vi "analyze magnet.vi"(0 "display queues":T3, 1 "disk queues":T3, 3 "trigger":bool, 4 "graph type":enum16{"absolute", "relative"}(ring), 5 "error in (no error)":errorcluster, 11 "toffset":dbl, 12 "crossing stats":T2) -> (10 "mag pos axes limits":cluster{"mag pos max":dbl, "mag pos min":dbl}, 14 "x-y magnet graph":cluster{sgl[], sgl[]}[](array[cluster]), 15 "magnet time graphs":cluster{dbl[], sgl[]}[](array[cluster]), 16 "fit parameters":T1, 19 "error out":errorcluster)   [LabVIEW 2017]
uses:
  typedefs/queue cluster.ctl
  typedefs/reading queue.ctl
  typedefs/reading.ctl
  typedefs/readingType.ctl
  typedefs/reading 1 queue.ctl
  typedefs/reading1.ctl
  typedefs/magnetic field fit.ctl
panel:
  in  "time range (s)":dbl=2.2 format="%#_13g"
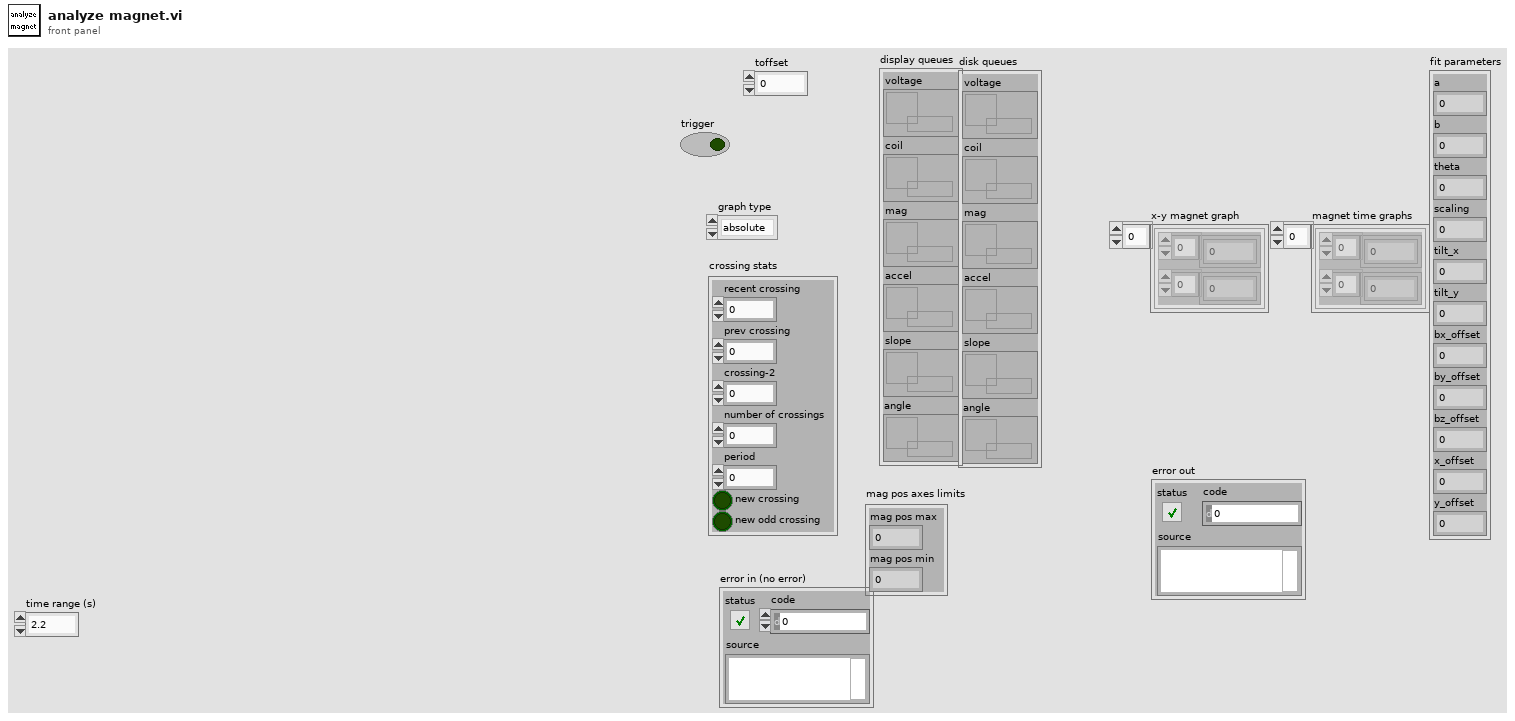
[diagram p1: front panel]
types:
  T1 = typedef "magnetic field fit.ctl" = cluster{"a":dbl, "b":dbl, "theta":dbl, "scaling":dbl, "tilt_x":dbl, "tilt_y":dbl, "bx_offset":dbl, "by_offset":dbl, "bz_offset":dbl, "x_offset":dbl, "y_offset":dbl}
  T2 = cluster{"recent crossing":dbl, "prev crossing":dbl, "crossing-2":dbl, "number of crossings":i32, "period":dbl, "new crossing":bool, "new odd crossing":bool}
  T3 = typedef "queue cluster.ctl" = cluster{"voltage":T4, "coil":T4, "mag":T4, "accel":T4, "slope":T5, "angle":T4}
  T4 = typedef "reading queue.ctl" = refnum<queue>
  T5 = typedef "reading 1 queue.ctl" = refnum<queue>
  T6 = typedef "reading.ctl" = cluster{"reading type":T7, "time":fxp<+,48,48>, "x":sgl, "y":sgl, "z":sgl, "XSUM":u8}
  T7 = typedef "readingType.ctl" = enum8{"SYNC", "DETVAL", "COILI", "MAGVEC", "ACCVEC"}
  T8 = cluster{"tx":cluster{dbl[], sgl[]}, "ty":cluster{dbl[], sgl[]}, "tz":cluster{dbl[], sgl[]}, "xy":cluster{sgl[], sgl[]}}
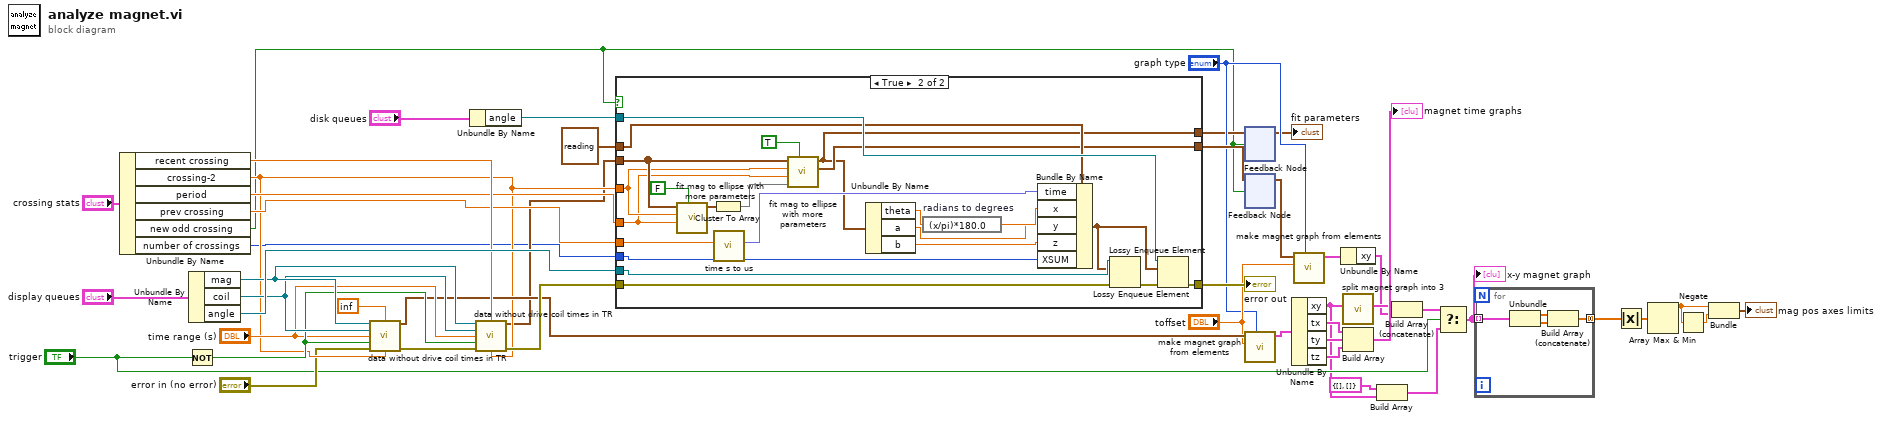
[diagram p0: block diagram]
diagram:
  n1 = Unbundle By Name("crossing stats") -> ("recent crossing"=w41:dbl, "crossing-2"=w31:dbl, "period"=w32:dbl, "prev crossing"=w33:dbl, "new odd crossing"=w16:bool, "number of crossings"=w3:i32)
  n2 = Not(x="trigger") -> (.not. x?=w38:bool)
  n3 = Unbundle By Name("display queues") -> ("mag"=w40:T4, "coil"=w39:T4, "angle"=w46:T4)
  n4 = call "data without drive coil times in TR.vi"("data"=w40, "t1"=inf, "coil"=w39, "recent interval"="time range (s)", "most recent?"=w38, "error in (no error)"="error in (no error)", "t0"=w31) -> ("data_no_coil"=w35:T6[], "error out"=w18:errorcluster)  [unwired: 6 in, 1 out]
  n5 = Unbundle By Name("disk queues") -> ("angle"=w42:T4)
  n6 = call "data without drive coil times in TR.vi"("data"=w40, "t1"=w41, "coil"=w39, "recent interval"="time range (s)", "most recent?"=w38, "error in (no error)"=w18, "t0"=w31) -> ("data_no_coil"=w30:T6[], "error out"=w44:errorcluster)  [unwired: 6 in, 1 out]
  n7 = case shown="True" w16 {
    tunnel: w46 -> [_ w72]
    tunnel: [w49 w69] -> w45
    tunnel: w44 -> [w49 w71]
    tunnel: w42 -> [_ w68]
    tunnel: T6 {"reading type"=enum."SYNC", "time"=0.0, "x"=0.0, "y"=0.0, "z"=0.0, "XSUM"=0} ("angle and time") -> [_ w67]
    tunnel: w33 -> [_ w64]
    tunnel: w32 -> [_ w53]
    tunnel: w31 -> [_ w54]
    tunnel: w30 -> [_ w55]
    tunnel: [_ w57] -> w29
    tunnel: [_ w56] -> w17
    tunnel: w3 -> [_ w62]
    frame False {
    }
    frame True {
      n8 = call "fit mag to ellipse with more parameters.vi"("advanced fit"=FALSE, "T"=w53, "t0"=w54, "mag no drive"=w55) -> ("fit parameters"=w52:T1)  [unwired: 5 in, 2 out]
      n9 = Cluster To Array(cluster=w52) -> (array=w51:dbl[])
      n10 = call "time s to us.vi"("time (s)"=w64) -> ("time (us)"=w63:fxp<+,48,48>)  [unwired: 10 in]
      n11 = call "fit mag to ellipse with more parameters.vi"("advanced fit"=TRUE, "starting parameters"=w51, "T"=w53, "t0"=w54, "mag no drive"=w55) -> ("fit magnetic field"=w57:T6[], "fit parameters"=w56:T1)  [unwired: 4 in, 1 out]
      n12 = Unbundle By Name(w56) -> ("theta"=w65:dbl, "a"=w60:dbl, "b"=w59:dbl)
      n13 = expression code="(x/pi)*180.0" "radians to degrees"(w65) -> (w61:dbl)
      n14 = Bundle By Name(cluster=w67, "time"=w63, "x"=w61, "y"=w60, "z"=w59, "XSUM"=w62) -> (w66:T6)
      n15 = Lossy Enqueue Element(queue=w72, element=w66, error in (no error)=w71) -> (error out=w70:errorcluster)  [unwired: 3 out]
      n16 = Lossy Enqueue Element(queue=w68, element=w66, error in (no error)=w70) -> (error out=w69:errorcluster)  [unwired: 3 out]
    }
  }
  "error out" <- w45
  n17 = feedback #1() -> (→"fit parameters":T1)  [unwired: 1 in]
  n18 = feedback-in #1(w17, w16) -> ()
  n19 = feedback-in #2(w29, w16) -> ()
  n20 = feedback #2() -> (w27:T6[])  [unwired: 1 in]
  n21 = call "make magnet graph from elements.vi"("graph type"="graph type", "toffset"="toffset", "elements"=w35) -> ("graphs"=w26:T8)  [unwired: 7 in, 1 out]
  n22 = Unbundle By Name(w26) -> ("xy"=w6:cluster{sgl[], sgl[]}, "tx"=w23:cluster{dbl[], sgl[]}, "ty"=w22:cluster{dbl[], sgl[]}, "tz"=w21:cluster{dbl[], sgl[]})
  n23 = call "make magnet graph from elements.vi"("graph type"="graph type", "toffset"="toffset", "elements"=w27) -> ("graphs"=w25:T8)  [unwired: 7 in, 1 out]
  n24 = Unbundle By Name(w25) -> ("xy"=w1:cluster{sgl[], sgl[]})
  n25 = call "split magnet graph into 3.vi"("graph in"=w6) -> ("graph array"=w8:cluster{sgl[], sgl[]}[])  [unwired: 10 in]
  n26 = Build Array(w23, w22, w21) -> (→"magnet time graphs":cluster{dbl[], sgl[]}[])
  n27 = Build Array(cluster{sgl[], sgl[]} {[], []} ("element"), w6) -> (w5:cluster{sgl[], sgl[]}[])
  n28 = Build Array (concatenate)(w8, w1) -> (w2:cluster{sgl[], sgl[]}[])
  n29 = Select(t=w2, s="trigger", f=w5) -> (s? t:f=w9:cluster{sgl[], sgl[]}[])
  "x-y magnet graph" <- w9
  n30 = for {
    tunnel: w9 -> [w76] mode=indexing
    tunnel: [w74] -> w12 mode=concatenating
    n31 = Unbundle(w76) -> (w75:sgl[], w73:sgl[])
    n32 = Build Array (concatenate)(w75, w73) -> (w74:sgl[])
  }
  n33 = Absolute Value(x=w12) -> (abs(x)=w11:sgl[])
  n34 = Array Max & Min(array=w11) -> (max value=w13:sgl)  [unwired: 3 out]
  n35 = Negate(x=w13) -> (-x=w14:sgl)
  n36 = Bundle(w13, w14) -> (→"mag pos axes limits":cluster{sgl, sgl})  [unwired: 1 in]
